vi "XYZAnalysis.vi"(0 "Reflectance":dbl[](array[numeric]), 1 "Illuminant":dbl[](array[numeric]), 2 "CMF":dbl[][](array[numeric])) -> ()   [LabVIEW 2013]
panel:
  out "Reflectance":cluster{dbl[], "Reflectance":dbl[]}(graph)
  out "Illuminant":cluster{dbl[], "Illuminant":dbl[]}(graph)
  out "Tristimulus":cluster{dbl[], "Reflectance":dbl[]}[](graph)
  out "XYZ x IS":cluster{dbl[], "Reflectance":dbl[]}[](graph)
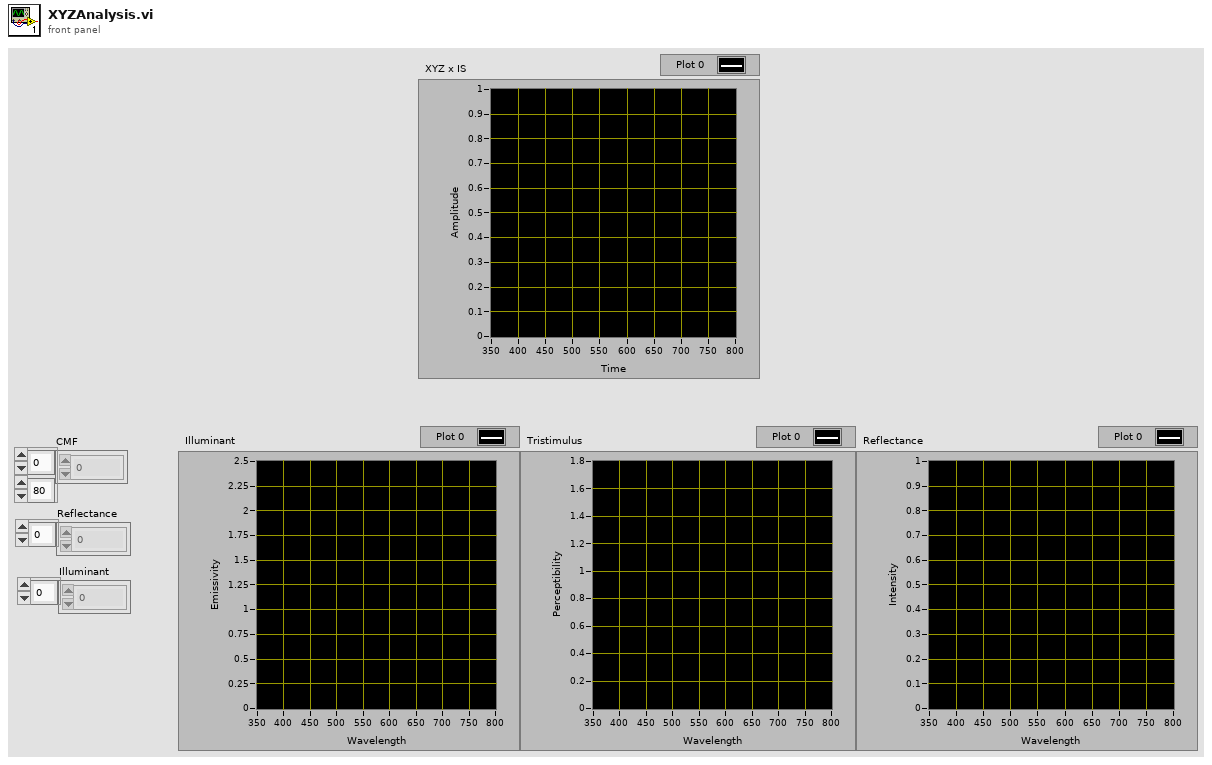
[diagram p1: front panel]
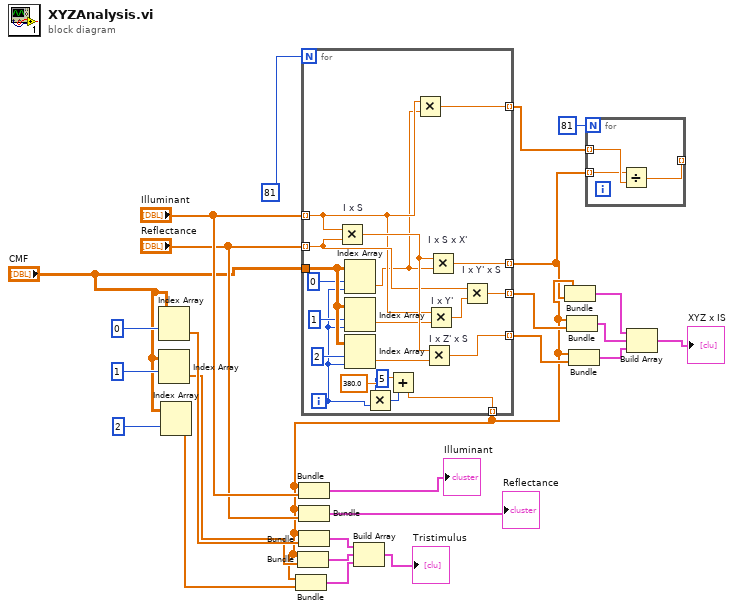
[diagram p0: block diagram]
diagram:
  n1 = Index Array(array="CMF", index (row)=0) -> (element=w17:dbl[])  [unwired: 1 in]
  n2 = Index Array(array="CMF", index (row)=1) -> (element=w16:dbl[])  [unwired: 1 in]
  n3 = Index Array(array="CMF", index (row)=2) -> (element=w15:dbl[])  [unwired: 1 in]
  n4 = for {
    N: 81 -> [_]
    tunnel: "CMF" -> [w46]
    tunnel: "Illuminant" -> [w30] mode=indexing
    tunnel: "Reflectance" -> [w43] mode=indexing
    tunnel: [w42] -> w19 mode=indexing
    tunnel: [w41] -> w4 mode=indexing
    tunnel: [w40] -> w18 mode=indexing
    tunnel: [w31] -> w5 mode=indexing
    tunnel: [w28] -> w6 mode=indexing
    i -> [w33]
    n5 = Multiply "I x S"(x=w30, y=w43) -> (x*y=w45:dbl)
    n6 = Index Array(array=w46, index (row)=0 ("disabled index (col)"), index (col)=w33) -> (element=w29:dbl)
    n7 = Index Array(array=w46, index (row)=1 ("disabled index (col)"), index (col)=w33) -> (element=w44:dbl)
    n8 = Index Array(array=w46, index (row)=2 ("disabled index (col)"), index (col)=w33) -> (element=w36:dbl)
    n9 = Multiply(x=5, y=w33) -> (x*y=w34:i32)
    n10 = Add(x=380.0, y=w34) -> (x+y=w31:dbl)
    n11 = Multiply(x=w30, y=w29) -> (x*y=w28:dbl)
    n12 = Multiply "I x Z' x S"(x=w45, y=w36) -> (x*y=w40:dbl)
    n13 = Multiply "I x Y'"(x=w30, y=w44) -> (x*y=w27:dbl)
    n14 = Multiply "I x S x X'"(x=w45, y=w29) -> (x*y=w41:dbl)
    n15 = Multiply "I x Y' x S"(x=w43, y=w27) -> (x*y=w42:dbl)
  }
  n16 = Bundle(w5, "CMF"=w15) -> (w12:cluster{dbl[], "CMF":dbl[]})  [unwired: 1 in]
  n17 = Bundle(w5, "CMF"=w16) -> (w13:cluster{dbl[], "CMF":dbl[]})  [unwired: 1 in]
  n18 = Bundle(w5, "Illuminant"="Illuminant") -> (→"Illuminant":cluster{dbl[], "Illuminant":dbl[]})  [unwired: 1 in]
  n19 = Bundle(w5, "Reflectance"="Reflectance") -> (→"Reflectance":cluster{dbl[], "Reflectance":dbl[]})  [unwired: 1 in]
  n20 = Bundle(w5, "CMF"=w17) -> (w14:cluster{dbl[], "CMF":dbl[]})  [unwired: 1 in]
  n21 = Build Array(w14, w13, w12) -> (→"Tristimulus":cluster{dbl[], "CMF":dbl[]}[])
  n22 = Bundle(w5, w4) -> (w23:cluster{dbl[], dbl[]})  [unwired: 1 in]
  n23 = Bundle(w5, w19) -> (w22:cluster{dbl[], dbl[]})  [unwired: 1 in]
  n24 = Bundle(w5, w18) -> (w21:cluster{dbl[], dbl[]})  [unwired: 1 in]
  n25 = for {
    N: 81 -> [_]
    tunnel: w6 -> [w48] mode=indexing
    tunnel: [w49] -> _ mode=indexing
    tunnel: w4 -> [w47] mode=indexing
    n26 = Divide(x=w47, y=w48) -> (x/y=w49:dbl)
  }
  n27 = Build Array(w23, w22, w21) -> (→"XYZ x IS":cluster{dbl[], dbl[]}[])
